vi "change device.vi"(5 "DeviceList":T2(array[cluster])) -> (2 "device":T1)   [LabVIEW 2020]
panel:
  in  "OK_Btn":bool
  in  "connected PQ-Laser Devices":u8(ring)
  # "Please choose a device and press OK:"
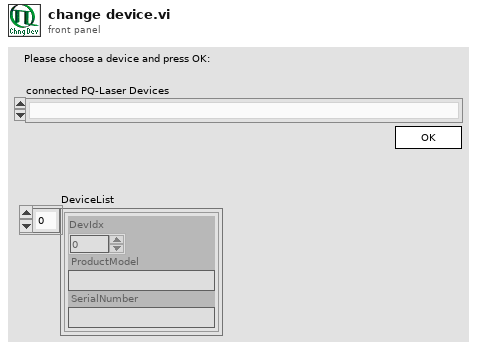
[diagram p1: front panel]
types:
  T1 = cluster{"DevIdx":i32, "ProductModel":string, "SerialNumber":string}
  T2 = cluster{"DevIdx":i32, "ProductModel":string, "SerialNumber":string}[]
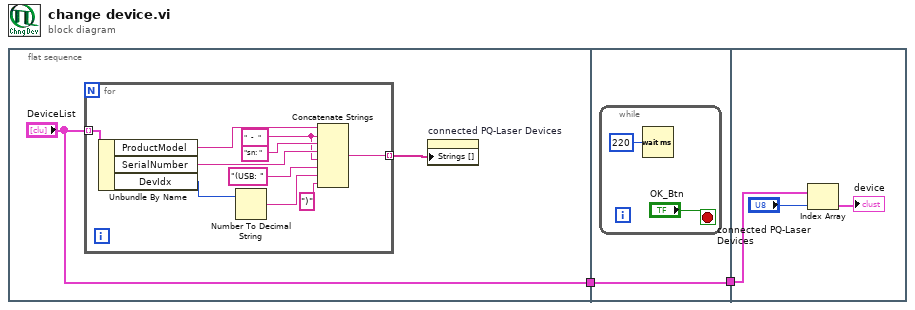
[diagram p0: block diagram]
diagram:
  n1 = flat-sequence {
    tunnel: ["DeviceList"] -> w1
    tunnel: [w15] -> w2
    tunnel: w1 -> [w15]
    tunnel: w2 -> [w19]
    frame #0 {
      n2 = for {
        tunnel: "DeviceList" -> [w14] mode=indexing
        tunnel: [w6] -> w4 mode=indexing
        w10 = "  -  " ("string")
        n3 = Unbundle By Name(w14) -> ("ProductModel"=w13:string, "SerialNumber"=w11:string, "DevIdx"=w5:i32)
        n4 = Number To Decimal String(number=w5) -> (decimal integer string=w7:string)  [unwired: 1 in]
        n5 = Concatenate Strings(w13, w10, "sn: " ("string"), w11, w10, "(USB: " ("string"), w7, ")" ("string")) -> (w6:string)
      }
      n6 = property on="connected PQ-Laser Devices" class="Ring (strict)"("Strings []"=w4) -> ()  [unwired: 2 in, 2 out]
    }
    frame #1 {
      n7 = while {
        stop <- "OK_Btn" stop-if-true
        n8 = Wait (ms)(milliseconds to wait=u32 220) -> ()  [unwired: 1 out]
      }
    }
    frame #2 {
      n9 = Index Array(array=w19, index="connected PQ-Laser Devices") -> (element=→"device":T1)
    }
  }
